vi "checkShutdown.vi"(8 "error in (no error)":errorcluster) -> (0 "error out":errorcluster, 3 "shutdown?":bool)   [LabVIEW 2018, in "TcpServer.lvclass"]
doc: "Check the Tcp Server shutdown request. Return a true boolean if yes."
uses:
  TcpServer.lvclass
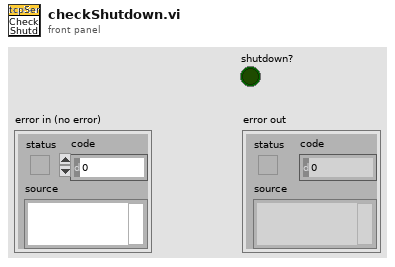
[diagram p1: front panel]
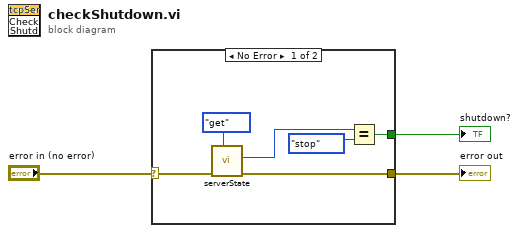
[diagram p0: block diagram]
diagram:
  n1 = case shown="No Error" "error in (no error)" {
    selector: "error in (no error)" -> [w9 w10]
    tunnel: [w8 w10] -> w2
    tunnel: [w5 _] -> w1
    frame No Error {
      n2 = call "serverState.vi"("function"=enum16{"set", "get"}."get", "error in (no error)"=w9) -> ("error out"=w8:errorcluster, "state"=w6:enum16{"stop", "run"})  [unwired: 8 in]
      n3 = Equal?(x=w6, y=enum16{"stop", "run"}."stop") -> (x = y?=w5:bool)
    }
    frame Error {
    }
  }
  "error out" <- w2
  "shutdown?" <- w1
